vi "TempFileCheck.vi"() -> (1 "파일수":u16, 3 "온도 파일 배열":string[](array[string]), 5 "연결된 문자열":string)   [LabVIEW 2020]
panel:
  out "파일 이름":string[](array[string])
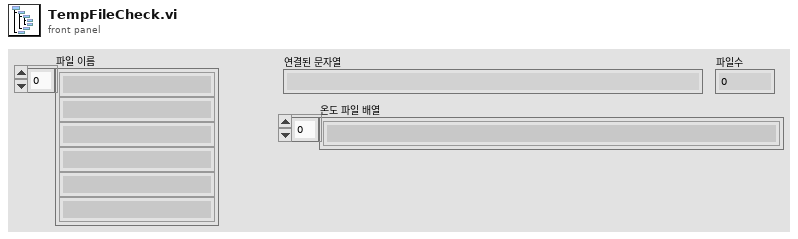
[diagram p1: front panel]
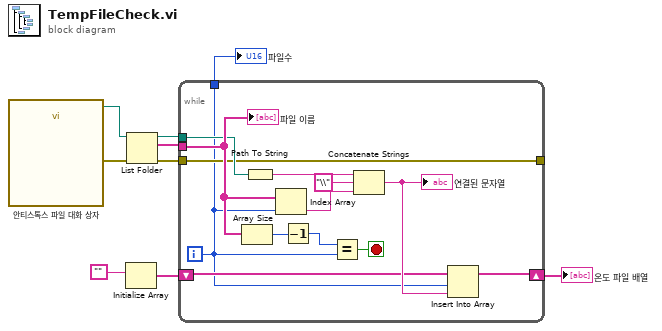
[diagram p0: block diagram]
diagram:
  n1 = call "안티스톡스 파일 대화 상자"() -> ("selected path"=w9:path, "error out"=w8:errorcluster)  [unwired: 12 in, 2 out]
  n2 = Initialize Array("") -> (w4:string[])  [unwired: 1 in]
  n3 = List Folder(path=w9, error in=w8) -> (path out=w7:path, filenames=w6:string[], error out=w2:errorcluster)  [unwired: 2 in, 1 out]
  n4 = while {
    tunnel: w7 -> [w14]
    tunnel: w6 -> [w18]
    shift-right: [w15] -> w3
    shift-left: w4 -> [w16]
    tunnel: [w13] -> _
    tunnel: w2 -> [w13]
    tunnel: [w10] -> w1
    i -> [w10]
    stop <- w19 stop-if-true
    n5 = Array Size(array=w18) -> (size(s)=w22:i32)
    n6 = Path To String(path=w14) -> (string=w21:string)
    n7 = Index Array(array=w18, index=w10) -> (element=w12:string)
    n8 = Decrement(x=w22) -> (x-1=w20:i32)
    n9 = Equal?(x=w20, y=w10) -> (x = y?=w19:bool)
    n10 = Concatenate Strings(w21, "\\", w12) -> (w17:string)
    "연결된 문자열" <- w17
    n11 = Insert Into Array(array=w16, index=w10, new element=w17) -> (w15:string[])
    "파일 이름" <- w18
  }
  "온도 파일 배열" <- w3
  "파일수" <- w1
